vi "allStatus.vi"(7 "all pos array 2":refnum<vi>, 10 "generic class reference":refnum<vi>, 11 "Array in":refnum<vi>) -> ()   [LabVIEW 2013]
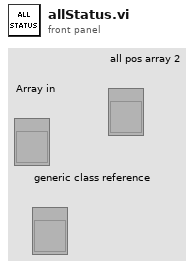
[diagram p1: front panel]
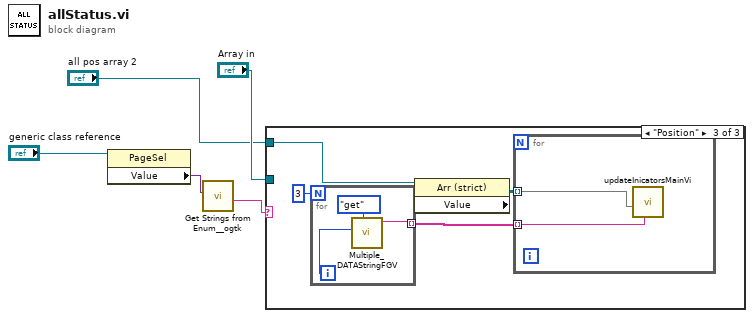
[diagram p0: block diagram]
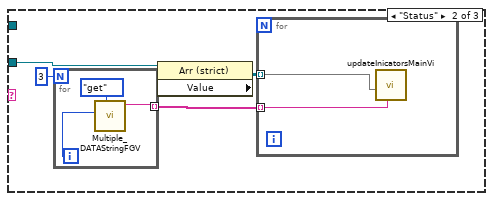
[diagram p3: hidden frame]
diagram:
  n1 = property class="PageSel"(reference="generic class reference") -> ("Value"=w2:variant)  [unwired: 1 in, 2 out]
  n2 = call <userlib>:"Get Strings from Enum__ogtk.vi"("Enum"=w2) -> ("String Value"=w1:string)  [unwired: 7 in, 3 out]
  n3 = case shown="\"Position\"" w1 {
    tunnel: "Array in" -> [_ w6 _]
    tunnel: "all pos array 2" -> [_ _ w15]
    frame "Main", Default {
    }
    frame "Status" {
      n4 = for {
        N: 3 -> [_]
        tunnel: [w12] -> w9 mode=indexing
        i -> [w13]
        n5 = call "Multiple_DATAStringFGV.vi"("Command"=enum16{"get", "set", "init"}."get", "Nr."=w13) -> ("Data String out"=w12:string)  [unwired: 9 in]
      }
      n6 = property class="Arr (strict)"(reference=w6) -> ("Value"=w8:refnum<vi>[][])  [unwired: 1 in, 2 out]
      n7 = for {
        tunnel: w8 -> [w11] mode=indexing
        tunnel: w9 -> [w10] mode=indexing
        n8 = call "updateInicatorsMainVi.vi"("Data String out"=w10, "Array"=w11) -> ()  [unwired: 7 in, 3 out]
      }
    }
    frame "Position" {
      n9 = for {
        N: 3 -> [_]
        tunnel: [w21] -> w18 mode=indexing
        i -> [w22]
        n10 = call "Multiple_DATAStringFGV.vi"("Command"=enum16{"get", "set", "init"}."get", "Nr."=w22) -> ("Data String out"=w21:string)  [unwired: 9 in]
      }
      n11 = property class="Arr (strict)"(reference=w15) -> ("Value"=w17:refnum<vi>[][])  [unwired: 1 in, 2 out]
      n12 = for {
        tunnel: w17 -> [w20] mode=indexing
        tunnel: w18 -> [w19] mode=indexing
        n13 = call "updateInicatorsMainVi.vi"("Data String out"=w19, "Array"=w20) -> ()  [unwired: 7 in, 3 out]
      }
    }
  }
